vi "BoxCrossPict.vi"(0 "Pict In":picture, 1 "rect":T1) -> (2 "Pict Out":picture, 3 "cursorX":i32, 4 "cursorY":i32)   [LabVIEW 2011]
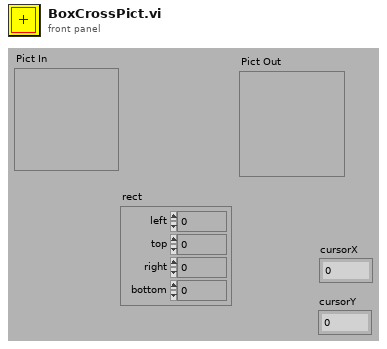
[diagram p1: front panel]
types:
  T1 = cluster{"left":i16, "top":i16, "right":i16, "bottom":i16}
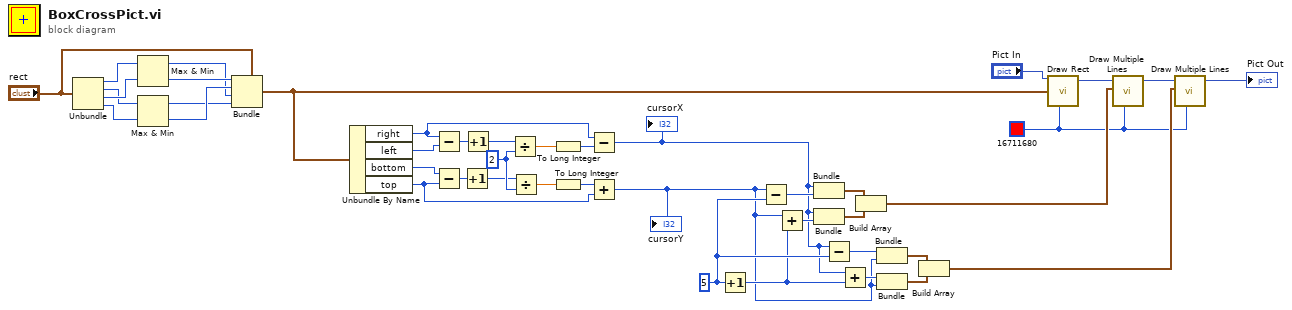
[diagram p0: block diagram]
diagram:
  w23 = 2
  w32 = 5
  w17 = u32 16711680
  n1 = Unbundle("rect") -> ("left"=w14:i16, "top"=w12:i16, "right"=w13:i16, "bottom"=w11:i16)
  n2 = Max & Min(x=w14, y=w13) -> (max(x,y)=w7:i16, min(x,y)=w8:i16)
  n3 = Max & Min(x=w12, y=w11) -> (max(x,y)=w9:i16, min(x,y)=w10:i16)
  n4 = Bundle(cluster="rect", "left"=w8, "top"=w10, "right"=w7, "bottom"=w9) -> (w5:T1)
  n5 = Unbundle By Name(w5) -> ("right"=w21:i16, "left"=w28:i16, "bottom"=w27:i16, "top"=w19:i16)
  n6 = Subtract(x=w21, y=w28) -> (x-y=w26:i16)
  n7 = Subtract(x=w27, y=w19) -> (x-y=w25:i16)
  n8 = Increment(x=w25) -> (x+1=w22:i16)
  n9 = Increment(x=w26) -> (x+1=w24:i16)
  n10 = Divide(x=w24, y=w23) -> (x/y=w3:dbl)
  n11 = Divide(x=w22, y=w23) -> (x/y=w4:dbl)
  n12 = To Long Integer(number=w3) -> (32bit integer=w20:i32)
  n13 = To Long Integer(number=w4) -> (32bit integer=w18:i32)
  n14 = Subtract(x=w21, y=w20) -> (x-y=w2:i32)
  "cursorX" <- w2
  n15 = Add(x=w18, y=w19) -> (x+y=w1:i32)
  "cursorY" <- w1
  n16 = Increment(x=w32) -> (x+1=w31:i32)
  n17 = Subtract(x=w1, y=w32) -> (x-y=w40:i32)
  n18 = Add(x=w1, y=w31) -> (x+y=w39:i32)
  n19 = Bundle(w2, w40) -> (w38:cluster{i32, i32})  [unwired: 1 in]
  n20 = Bundle(w2, w39) -> (w37:cluster{i32, i32})  [unwired: 1 in]
  n21 = Subtract(x=w2, y=w32) -> (x-y=w33:i32)
  n22 = Add(x=w2, y=w31) -> (x+y=w34:i32)
  n23 = Build Array(w38, w37) -> (w30:cluster{i32, i32}[])
  n24 = Bundle(w33, w1) -> (w35:cluster{i32, i32})  [unwired: 1 in]
  n25 = Bundle(w34, w1) -> (w36:cluster{i32, i32})  [unwired: 1 in]
  n26 = Build Array(w35, w36) -> (w29:cluster{i32, i32}[])
  n27 = call <vilib>:"Draw Rect.vi"("picture"="Pict In", "rect"=w5, "color(black)"=w17) -> ("new picture"=w41:picture)  [unwired: 6 in]
  n28 = call <vilib>:"Draw Multiple Lines.vi"("picture"=w41, "line endpoints"=w30, "color(black)"=w17) -> ("new picture"=w42:picture)  [unwired: 6 in]
  n29 = call <vilib>:"Draw Multiple Lines.vi"("picture"=w42, "line endpoints"=w29, "color(black)"=w17) -> ("new picture"=→"Pict Out":picture)  [unwired: 6 in]
